vi "SavePassSettings.vi"(11 "notifier":refnum<notifier>) -> ()   [LabVIEW 2013, in "main.lvlib"]
uses:
  main.lvlib
panel:
  in  "invalidPassStr":string="Kodeord ugyldigt"
  in  "incompPassStr":string="Kodeord ikke ens"
  in  "SaveBtn":bool
  out "presentPassValidationStr":string caption="OkStr 2"
  out "newPassValidationStr":string caption="OkStr"
  in  "NewPassword":string caption="Nyt Kodeord"
  in  "RetypePassword":string caption="Gentag"
  in  "PresentPassword":string caption="Nuværende Kodeord"
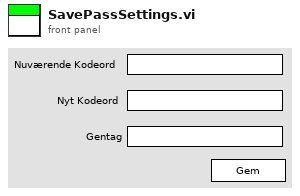
[diagram p1: front panel]
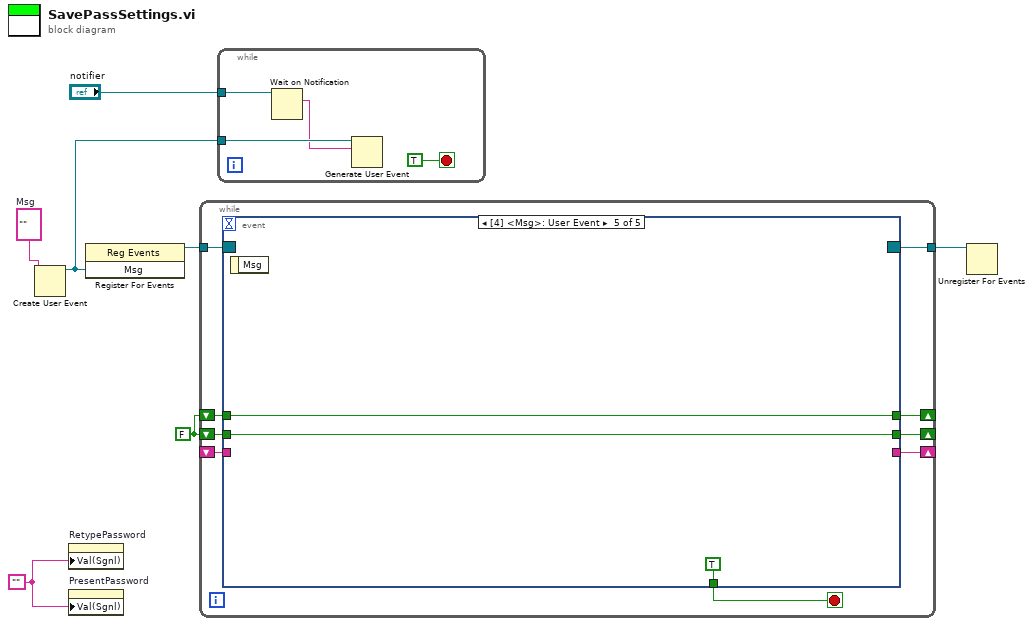
[diagram p0: block diagram]
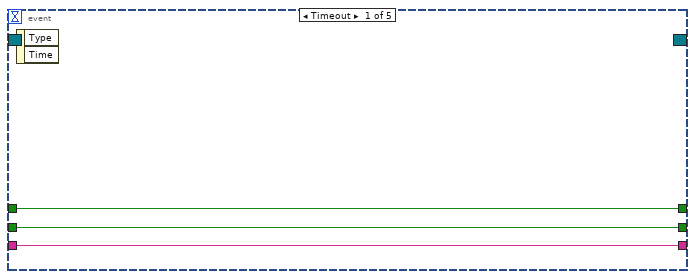
[diagram p2: hidden frame]
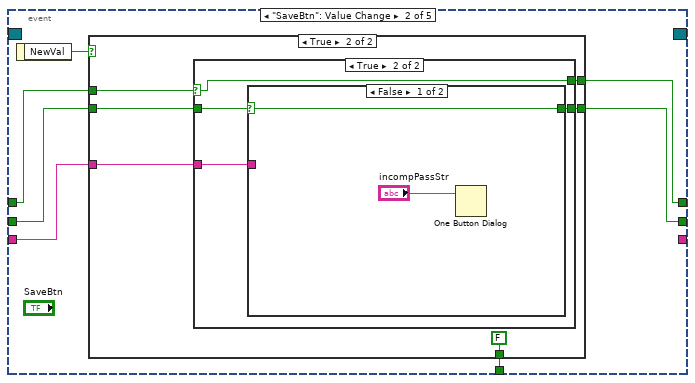
[diagram p3: hidden frame]
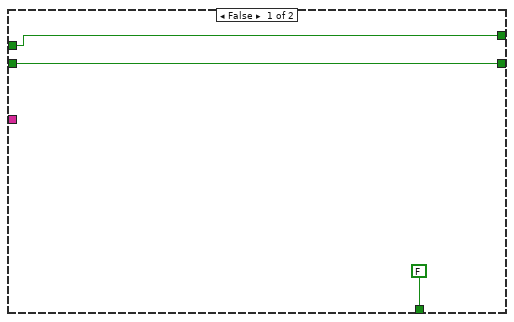
[diagram p4: hidden frame]
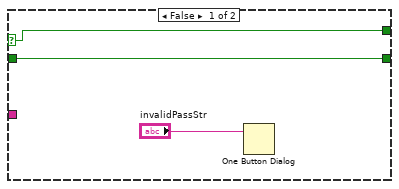
[diagram p5: hidden frame]
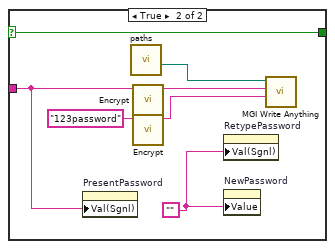
[diagram p6: hidden frame]
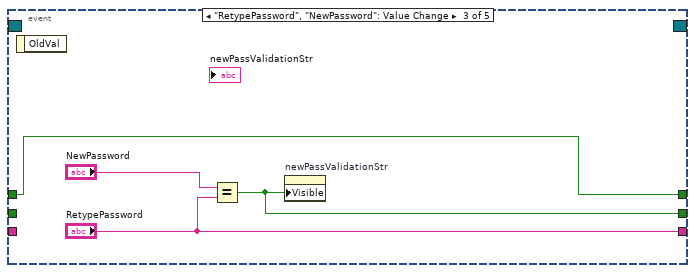
[diagram p7: hidden frame]
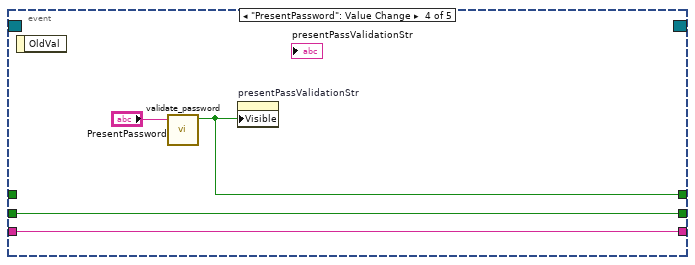
[diagram p8: hidden frame]
diagram:
  w2 = ""
  w3 = FALSE
  w5 = ""  # Msg
  n1 = Create User Event(user event datatype=w5) -> (user event=w4:refnum<user-event>)  [unwired: 1 in, 1 out]
  n2 = property on="RetypePassword" class="Str"("Val(Sgnl)"=w2) -> ()  [unwired: 2 in, 2 out]
  n3 = property on="PresentPassword" class="Str"("Val(Sgnl)"=w2) -> ()  [unwired: 2 in, 2 out]
  n4 = register-events(w4) -> (reference out=w6:refnum<event-registration>)  [unwired: 2 in, 1 out]
  n5 = while {
    tunnel: w6 -> [w16]
    shift-right: [w14] -> _
    shift-left: _ -> [w11]
    shift-right: [w13] -> _
    shift-left: w3 -> [w12]
    shift-right: [w10] -> _
    shift-left: w3 -> [w9]
    tunnel: [w8] -> w1
    stop <- w15 stop-if-true
    n6 = event shown="[4] <Msg>: User Event" {
      selector: w16 -> [_ _ _ _ _]
      dyn-events: [_ _ _ _ _] -> w8
      timeout: _ -> [_ _ _ _ _]
      tunnel: [_ w26 _ _ TRUE] -> w15
      tunnel: [w18 _ "RetypePassword" w57 _] -> w14
      tunnel: [w19 w21 w53 w58 w61] -> w13
      tunnel: w12 -> [w19 w25 _ w58 w61]
      tunnel: w11 -> [w18 w24 _ w57 _]
      tunnel: [w17 w20 w52 w56 w60] -> w10
      tunnel: w9 -> [w17 w23 w52 _ w60]
      event Timeout {
        n7 = event-data() -> ()  [unwired: 1 in, 2 out]
      }
      event "SaveBtn": Value Change {
        n8 = event-data() -> ("NewVal"=w22:bool)  [unwired: 1 in]
        n9 = case shown="True" w22 {
          tunnel: [FALSE FALSE] -> w26
          tunnel: w25 -> [w27 w34]
          tunnel: w24 -> [_ w33]
          tunnel: w23 -> [w28 w32]
          tunnel: [w27 w31] -> w21
          tunnel: [w28 w30] -> w20
          frame False {
          }
          frame True {
            n10 = case shown="True" w32 {
              selector: w32 -> [w37 w39]
              tunnel: w34 -> [w36 w42]
              tunnel: w33 -> [_ w41]
              tunnel: [w36 w40] -> w31
              tunnel: [w37 w39] -> w30
              frame False {
                n11 = One Button Dialog(message="invalidPassStr") -> ()  [unwired: 1 in, 1 out]
              }
              frame True {
                n12 = case shown="False" w42 {
                  selector: w42 -> [w43 w45]
                  tunnel: w41 -> [_ w46]
                  tunnel: [w43 w45] -> w40
                  frame False {
                    n13 = One Button Dialog(message="incompPassStr") -> ()  [unwired: 1 in, 1 out]
                  }
                  frame True {
                    w47 = ""
                    n14 = property on="PresentPassword" class="Str"("Val(Sgnl)"=w46) -> ()  [unwired: 2 in, 2 out]
                    n15 = call "paths.vi"() -> ("Controlsettings2"=w48:path)  [unwired: 8 in, 3 out]
                    n16 = call "Encrypt.vi"("Input"=w46) -> ("Output"=w49:string)  [unwired: 10 in]
                    n17 = call "Encrypt.vi"("Input"="123password") -> ("Output"=w50:string)  [unwired: 10 in]
                    n18 = property on="RetypePassword" class="Str"("Val(Sgnl)"=w47) -> ()  [unwired: 2 in, 2 out]
                    n19 = property on="NewPassword" class="Str"("Value"=w47) -> ()  [unwired: 2 in, 2 out]
                    n20 = call <userlib>:"MGI Write Anything.vi"("Section Name (Name of \"Anything\")"=w50, "Anything"=w49, "Path (dialog)"=w48) -> ()  [unwired: 6 in, 3 out]
                  }
                }
              }
            }
          }
        }
      }
      event "RetypePassword", "NewPassword": Value Change {
        n21 = event-data() -> ()  [unwired: 1 in, 1 out]
        n22 = Equal?(x="NewPassword", y="RetypePassword") -> (x = y?=w53:bool)
        n23 = property on="newPassValidationStr" class="Str"("Visible"=w53) -> ()  [unwired: 2 in, 2 out]
      }
      event "PresentPassword": Value Change {
        n24 = event-data() -> ()  [unwired: 1 in, 1 out]
        n25 = call "validate_password.vi"("Password"="PresentPassword") -> ("Accept"=w56:bool)  [unwired: 10 in]
        n26 = property on="presentPassValidationStr" class="Str"("Visible"=w56) -> ()  [unwired: 2 in, 2 out]
      }
      event User Event {
        n27 = event-data() -> ()  [unwired: 1 in, 1 out]
      }
    }
  }
  n28 = while {
    tunnel: "notifier" -> [w66]
    tunnel: w4 -> [w64]
    stop <- TRUE stop-if-true
    n29 = Wait on Notification(notifier=w66) -> (notification=w63:string)  [unwired: 3 in, 3 out]
    n30 = Generate User Event(user event=w64, event data cluster=w63) -> ()  [unwired: 2 in, 2 out]
  }
  n31 = Unregister For Events(event registration refnum=w1) -> ()  [unwired: 1 in, 1 out]
